vi "RemoveCharacters.vi"(1 "first row":string[](array[string])) -> (0 "Array":string[](array[string]))   [LabVIEW 2019, in "VCL_2_DSC.lvclass"]
uses:
  VCL_2_DSC.lvclass
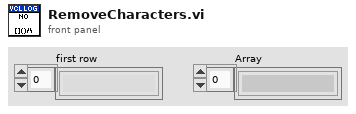
[diagram p1: front panel]
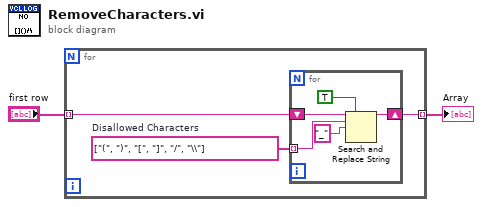
[diagram p0: block diagram]
diagram:
  n1 = for {
    tunnel: "first row" -> [w4] mode=indexing
    tunnel: [w3] -> w2 mode=indexing
    w5 = string[] ["(", ")", "[", "]", "/", "\\"]  # Disallowed Characters
    n2 = for {
      tunnel: w5 -> [w8] mode=indexing
      shift-right: [w6] -> w3
      shift-left: w4 -> [w9]
      n3 = Search and Replace String(replace all?=TRUE ("replace all? (F)"), input string=w9, search string=w8, replace string="_" ("replace string (\"\")")) -> (result string=w6:string)  [unwired: 4 in, 3 out]
    }
  }
  "Array" <- w2
